vi "Logging Unsplit Path.vi"(1 "Split Path":string[](array[string])) -> (0 "Path":string)   [LabVIEW 2012, in "femtoRoboLib.lvlib"]
uses:
  femtoRoboLib.lvlib
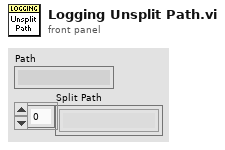
[diagram p1: front panel]
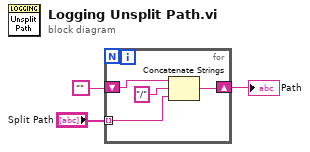
[diagram p0: block diagram]
diagram:
  n1 = for {
    tunnel: "Split Path" -> [w5] mode=indexing
    shift-right: [w4] -> w1
    shift-left: "" -> [w7]
    n2 = Concatenate Strings(w7, "/" ("string"), w5) -> (w4:string)
  }
  "Path" <- w1
